vi "LV86_Get Pixel Value.vi"(4 "Position":cluster{"X":u32, "Y":u32}, 5 "Image In":T1 {"Dialogs" format="%.0b"}) -> (0 "RGB":cluster{"R":u32, "G":u32, "B":u32} {"B" format="%.0x"; "G" format="%.0x"; "R" format="%.0x"}, 1 "I":u32 format="%.0x", 2 "Image Out":T1 {"Dialogs" format="%.0b"})   [LabVIEW 2024]
doc: "This VI gets the value of the pixel located at the specified <B>Position</B> and returns its value (either as an 8-bit number or an <B>RGB</B> cluster)."
uses:
  <userlib>/ImageProcessing/QTLIB_2595_LV86/QT_Image.ctl
panel:
  # "This VI gets the value of the pixel located at the specified \nPosition and returns its value (either as an 8-bit \nnumber or an RGB cluster)."
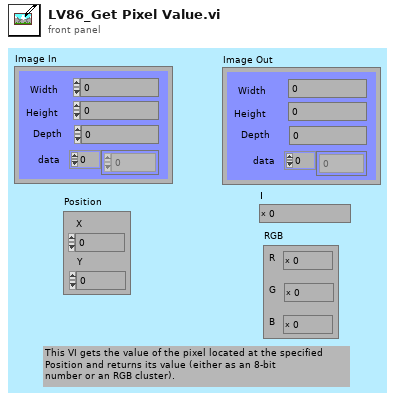
[diagram p1: front panel]
types:
  T1 = typedef "QT_Image.ctl" = cluster{"Width":i32, "Height":i32, "Depth":i32, "data":u8[], "Compressed data":u8[], "Color table":u32[], "Duration":i32, "Options":i32, "Timestamp":i32, "ID":i32, "Reserved":i32, "Dialogs":u32}
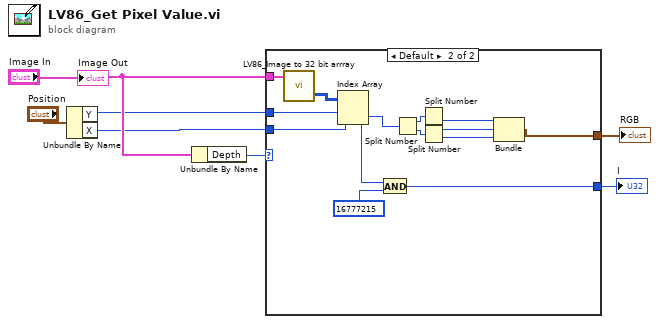
[diagram p0: block diagram]
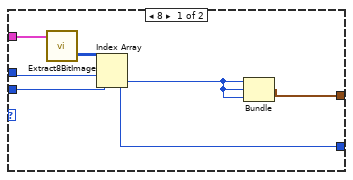
[diagram p2: hidden frame]
diagram:
  n1 = Unbundle By Name("Position") -> ("Y"=w4:u32, "X"=w3:u32)
  n2 = Unbundle By Name("Image In") -> ("Depth"=w6:i32)
  n3 = case shown="Default" w6 {
    tunnel: "Image In" -> [w13 w24]
    tunnel: w4 -> [w11 w23]
    tunnel: w3 -> [w10 w22]
    tunnel: [w9 w15] -> w2
    tunnel: [w8 w14] -> w1
    frame 8 {
      n4 = call <userlib>:"Extract8BitImage.vi"("Image in"=w13) -> ("Intensity Graph"=w12:u8[][])  [unwired: 1 in, 1 out]
      n5 = Index Array(array=w12, index (row)=w11, index (col)=w10) -> (element=w9:u8)
      n6 = Bundle(w9, w9, w9) -> (w8:cluster{u8, u8, u8})  [unwired: 1 out]
    }
    frame Default {
      n7 = call <userlib>:"LV86_Image to 32 bit arrray.vi"("Image In"=w24) -> ("Intensity Graph"=w25:u32[][])  [unwired: 1 in, 1 out]
      n8 = Index Array(array=w25, index (row)=w23, index (col)=w22) -> (element=w16:u32)
      n9 = And(x=w16, y=u32 16777215 ("hi")) -> (x .and. y?=w15:u32)
      n10 = Split Number(x=w16) -> (hi(x)=w21:u16, lo(x)=w26:u16)
      n11 = Split Number(x=w21) -> (lo(x)=w20:u8)  [unwired: 1 out]
      n12 = Split Number(x=w26) -> (hi(x)=w19:u8, lo(x)=w18:u8)
      n13 = Bundle(w20, w19, w18) -> (w14:cluster{u8, u8, u8})  [unwired: 1 out]
    }
  }
  "I" <- w2
  "RGB" <- w1
  "Image Out" <- "Image In"
